vi "Escribir TDMS Parametros Inversor.vi"(7 "semaphore":T1, 8 "error in":errorcluster, 9 "queue":refnum<queue>) -> (0 "error out":errorcluster, 1 "queue out":refnum<queue>, 2 "tdms sinc out":refnum<k34>, 3 "tdms historico out":refnum<k34>, 5 "semaphore out":T1)   [LabVIEW 2015]
uses:
  Application/ClusterM2.ctl
panel:
  out "M2":T2
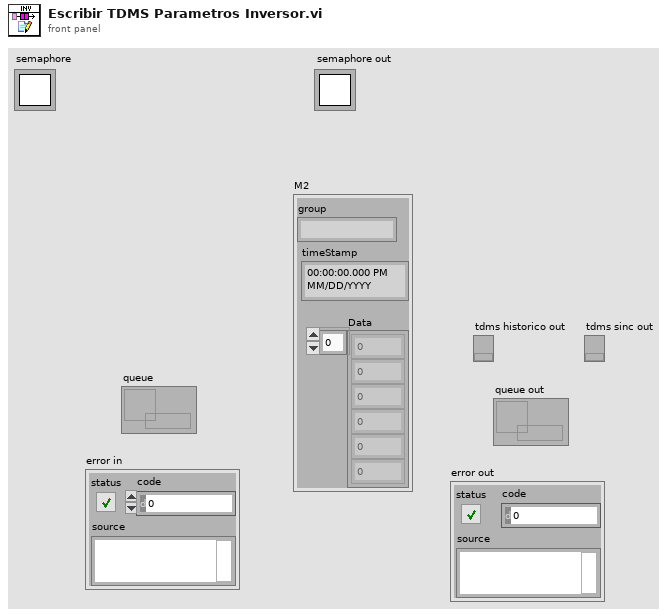
[diagram p1: front panel]
types:
  T1 = typedef "Semaphore RefNum" = refnum<k1>
  T2 = typedef "ClusterM2.ctl" = cluster{"timeStamp":timestamp, "Data":dbl[], "group":string}
  T3 = cluster{"tdms control out":refnum<k34>, "tdms historial out":refnum<k34>, "tdms sinc out":refnum<k34>}
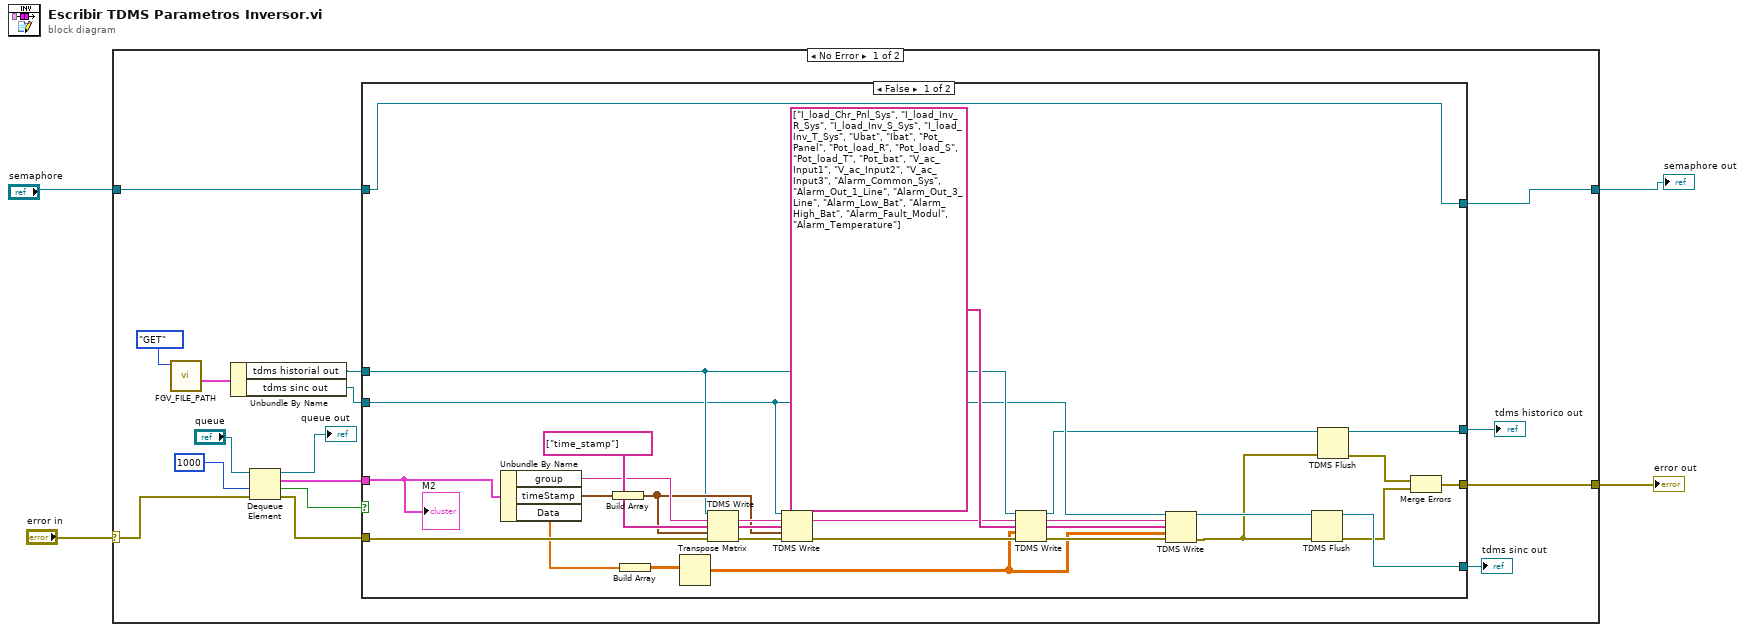
[diagram p0: block diagram]
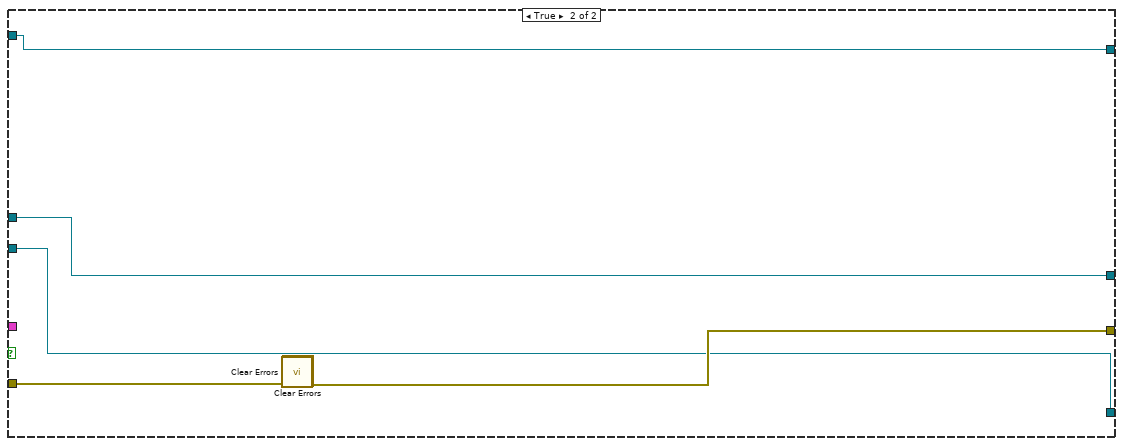
[diagram p2: hidden frame]
diagram:
  n1 = case shown="No Error" "error in" {
    selector: "error in" -> [w9 w56]
    tunnel: [w8 w56] -> w3
    tunnel: "semaphore" -> [w6 w55]
    tunnel: [w5 w55] -> w1
    frame No Error {
      n2 = call "FGV_FILE_PATH.vi"("Function"=enum16{"GET", "SET"}."GET") -> ("Data Out"=w7:T3)  [unwired: 10 in]
      n3 = Unbundle By Name(w7) -> ("tdms historial out"=w11:refnum<k34>, "tdms sinc out"=w10:refnum<k34>)
      n4 = Dequeue Element(queue="queue", timeout in ms (-1)=1000, error in (no error)=w9) -> (queue out=→"queue out":refnum<queue>, element=w19:T2, timed out?=w20:bool, error out=w18:errorcluster)
      n5 = case shown="False" w20 {
        tunnel: w19 -> [w47 _]
        tunnel: w18 -> [w46 w50]
        tunnel: [w21 w54] -> w8
        tunnel: w11 -> [w39 w53]
        tunnel: [w25 w52] -> w15
        tunnel: w10 -> [w36 w52]
        tunnel: [w27 w53] -> w13
        tunnel: [w29 w51] -> w5
        tunnel: w6 -> [w29 w51]
        frame False {
          n6 = Unbundle By Name(w47) -> ("group"=w44:string, "timeStamp"=w48:timestamp, "Data"=w32:dbl[])
          n7 = Build Array(w48) -> (w41:timestamp[])
          n8 = Build Array(w32) -> (w31:dbl[][])
          n9 = Transpose Matrix(1:w31) -> (0:w30:dbl[][])
          n10 = TDMS Write(0:w39, 5:w44, 7:string[] ["time_stamp"] ("channel name(s) in (Untitled)"), 9:w41, 11:w46) -> (6:w43:string, 8:w42:string[], 15:w40:errorcluster)  [unwired: 1 in, 1 out]
          n11 = TDMS Write(0:w36, 5:w43, 7:w42, 9:w41, 11:w40) -> (6:w38:string, 15:w37:errorcluster)  [unwired: 1 in, 2 out]
          n12 = TDMS Write(0:w39, 5:w38, 7:string[] ["I_load_Chr_Pnl_Sys", "I_load_Inv_R_Sys", "I_load_Inv_S_Sys", "I_load_Inv_T_Sys", "Ubat", "Ibat", "Pot_Panel", "Pot_load_R", "Pot_load_S", "Pot_load_T", "Pot_bat", "V_ac_Input1", "V_ac_Input2", "V_ac_Input3", "Alarm_Common_Sys", "Alarm_Out_1_Line", "Alarm_Out_3_Line", "Alarm_Low_Bat", "Alarm_High_Bat", "Alarm_Fault_Modul", "Alarm_Temperature"], 9:w30, 11:w37) -> (4:w28:refnum<k34>, 6:w35:string, 8:w34:string[], 15:w33:errorcluster)  [unwired: 1 in]
          n13 = TDMS Write(0:w36, 5:w35, 7:w34, 9:w30, 11:w33) -> (4:w26:refnum<k34>, 15:w23:errorcluster)  [unwired: 1 in, 2 out]
          n14 = TDMS Flush(4:w23, 7:w26) -> (0:w22:errorcluster, 3:w25:refnum<k34>)
          n15 = TDMS Flush(4:w23, 7:w28) -> (0:w24:errorcluster, 3:w27:refnum<k34>)
          n16 = Merge Errors(w24, w22) -> (w21:errorcluster)
          "M2" <- w47
        }
        frame True {
          n17 = call <vilib>:"Clear Errors.vi"() -> ("error out"=w54:errorcluster)  [unwired: 6 in, 1 out]
          n18 = call <vilib>:"Clear Errors.vi"("error in (no error)"=w50) -> ()  [unwired: 5 in, 2 out]
        }
      }
      "tdms sinc out" <- w15
      "tdms historico out" <- w13
    }
    frame Error {
    }
  }
  "error out" <- w3
  "semaphore out" <- w1
